vi "习 公式节点.vi"() -> ()   [LabVIEW 2017]
panel:
  out "波形图":dbl[](graph)
  in  "b":dbl
  in  "a":dbl
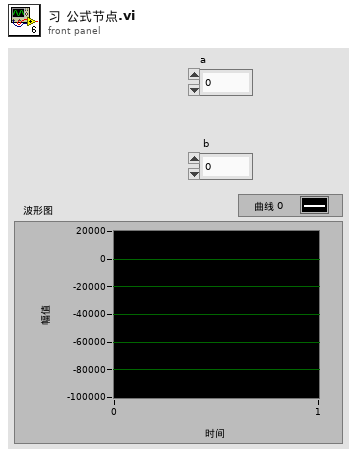
[diagram p1: front panel]
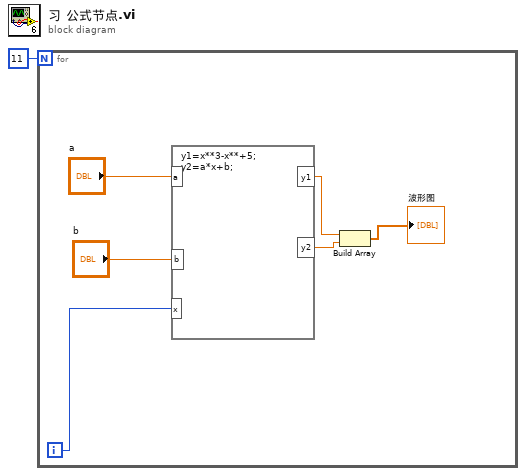
[diagram p0: block diagram]
diagram:
  n1 = for {
    N: 11 -> [_]
    i -> [w2]
    n2 = formula code="y1=x**3-x**+5;\ny2=a*x+b;"("a"="a", "b"="b", "x"=w2) -> ("y1"=w5:dbl, "y2"=w4:dbl)
    n3 = Build Array(w5, w4) -> (→"波形图":dbl[])
  }
